vi "Gen Library.vi"(8 "error in (no error)":errorcluster) -> (0 "error out":errorcluster)   [LabVIEW 2020, in "WebServiceImporter.lvlib" / "VI Generator.lvlib"]
uses:
  <vilib>/Platform/WebService/VI Generator/VI Generator.lvlib
  <vilib>/Platform/WebService/Error Handling/Error/Context Name.ctl
  <vilib>/Platform/WebService/Error Handling/Error/Error Number.ctl
  <vilib>/Platform/WebService/Error Handling/Error Handling.lvlib
  <resource>/importtools/Common/LabVIEW Library/NISAST LabVIEW Library.lvlib
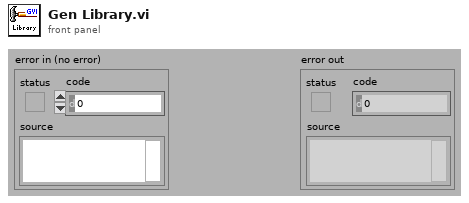
[diagram p1: front panel]
types:
  T1 = typedef "WebServiceImporter.lvlib/Error Handling.lvlib/Error Number.ctl" = u16
  T2 = typedef "WebServiceImporter.lvlib/Error Handling.lvlib/Context Name.ctl" = u16
  T3 = typedef "WebServiceImporter.lvlib/Error Handling.lvlib/Context.ctl" = cluster{"name":T2, "value":string}[]
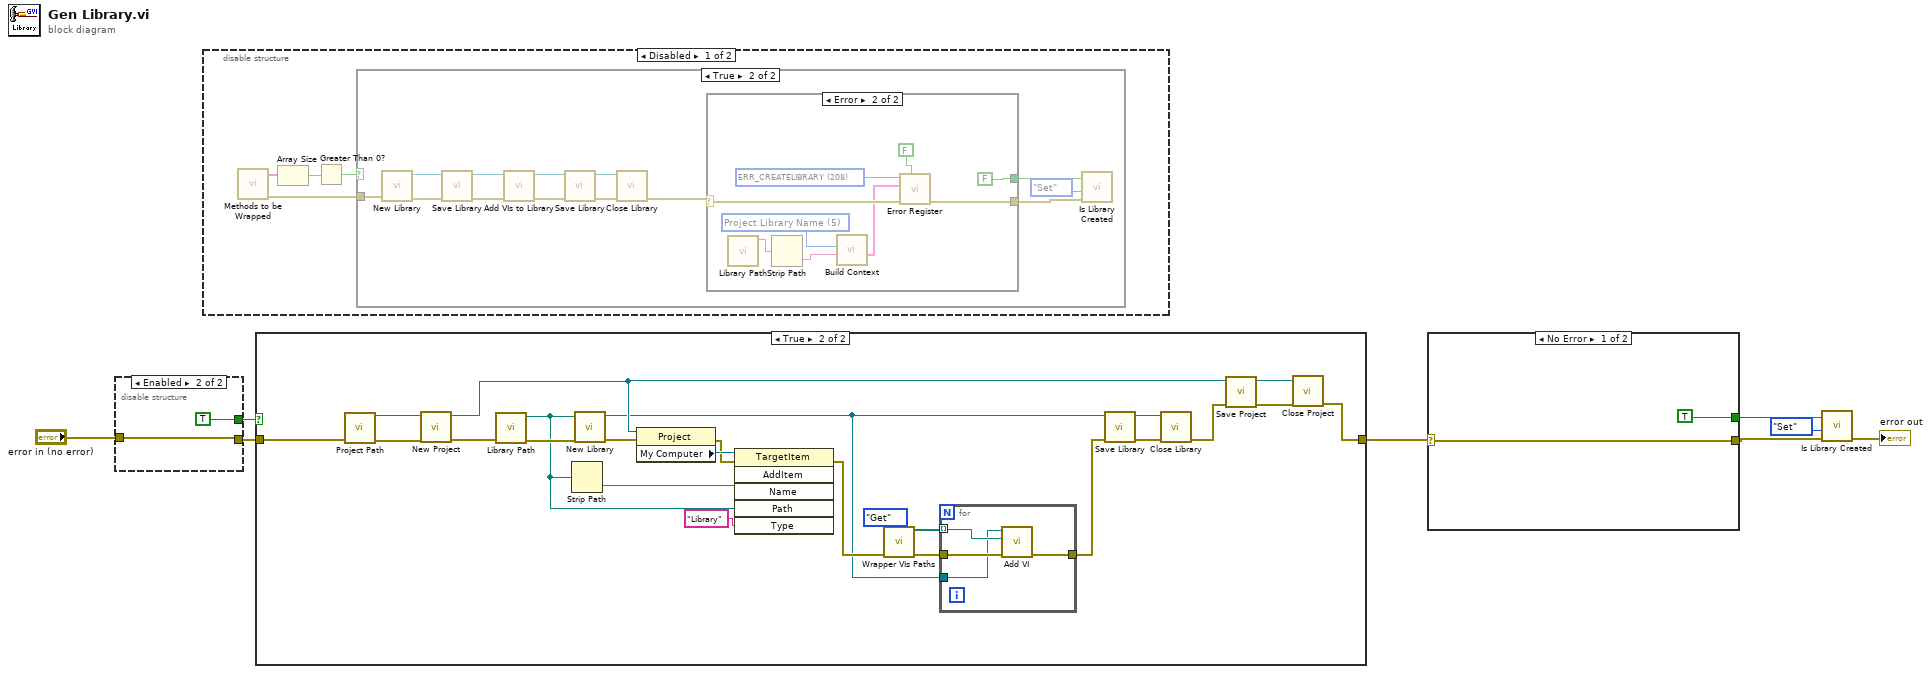
[diagram p0: block diagram]
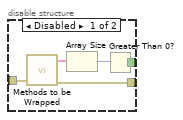
[diagram p2: hidden frame]
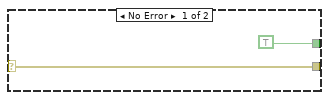
[diagram p4: hidden frame]
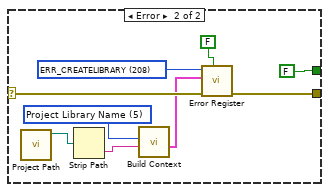
[diagram p6: hidden frame]
diagram:
  n1 = disable-structure shown="Enabled" {
    disable-tunnel: "error in (no error)" -> [w11 w15]
    disable-tunnel: [w10 TRUE] -> w7
    disable-tunnel: [w9 w15] -> w6
    frame Disabled {
      n2 = call <vilib>:"Methods to be Wrapped.vi"("error in (no error)"=w11) -> ("error out"=w9:errorcluster, "Methods to be Wrapped (out)"=w13:string[])  [unwired: 9 in]
      n3 = Array Size(array=w13) -> (size(s)=w12:i32)
      n4 = Greater Than 0?(x=w12) -> (x > 0?=w10:bool)
    }
    frame Enabled {
    }
  }
  n5 = disable-structure shown="Disabled" {
    frame Disabled {
      n6 = call <vilib>:"Methods to be Wrapped.vi"() -> ("error out"=w19:errorcluster, "Methods to be Wrapped (out)"=w16:string[])  [unwired: 10 in]
      n7 = Array Size(array=w16) -> (size(s)=w17:i32)
      n8 = Greater Than 0?(x=w17) -> (x > 0?=w18:bool)
      n9 = case shown="True" w18 {
        tunnel: w19 -> [_ w29]
        frame False {
        }
        frame True {
          n10 = call <vilib>:"New Library.vi"("error in (no error)"=w29) -> ("error out"=w23:errorcluster, "Library:Create"=w21:refnum<vi>)  [unwired: 9 in]
          n11 = call <vilib>:"Save Library.vi"("error in (no error)"=w23, "library"=w21) -> ("error out"=w22:errorcluster, "library out"=w20:refnum<vi>)  [unwired: 8 in]
          n12 = call <vilib>:"Add VIs to Library.vi"("error in"=w22, "Library"=w20) -> ("error out"=w32:errorcluster, "Library out"=w31:refnum<vi>)  [unwired: 8 in]
          n13 = call <vilib>:"Save Library.vi"("error in (no error)"=w32, "library"=w31) -> ("error out"=w25:errorcluster, "library out"=w30:refnum<vi>)  [unwired: 8 in]
          n14 = call <vilib>:"Close Library.vi"("error in (no error)"=w25, "library"=w30) -> ("error out"=w24:errorcluster)  [unwired: 9 in]
          n15 = case shown="Error" w24 {
            selector: w24 -> [w33 w39]
            tunnel: [TRUE FALSE] -> w27
            tunnel: [w33 w36] -> w26
            frame No Error {
            }
            frame Error {
              w37 = T1 208 items=["ERR_NOERROR"=0, "ERR_ACCESS_OUTPUTFOLDER"=1, "ERR_INVALID_LIBRARYNAME"=2, "ERR_CREATE_VIWRAPPER"=3, "ERR_UNKNOWN"=201, "ERR_BAD_ARGUMENT"=202, "ERR_URL_NOTFOUND_BADWSDL"=203, "ERR_BADLYFORMATTEDURL"=204, "ERR_BADHOSTNAME"=205, "ERR_BADDIRECTORY"=206, "ERR_UNAUTHORIZEDACCESS"=207, "ERR_CREATELIBRARY"=208] ("Error Number")
              w42 = T2 5 items=["Method Name", "Parameter Name", "VI Name", "Control Name", "Proxy Dll Path", "Project Library Name"] ("Context Name")
              n16 = call <vilib>:"Library Path.vi"() -> ("Path (out)"=w41:path)  [unwired: 10 in, 1 out]
              n17 = Strip Path(path=w41) -> (name=w40:string)  [unwired: 1 out]
              n18 = call <vilib>:"Build Context.vi"("Context Value"=w40, "Context Name"=w42) -> ("Context"=w38:T3)  [unwired: 9 in]
              n19 = call <vilib>:"Error Register.vi"("Throw Up?"=FALSE, "error in (no error)"=w39, "Context"=w38, "Error Number"=w37) -> ("error out"=w36:errorcluster)  [unwired: 7 in]
            }
          }
          n20 = call <vilib>:"Is Library Created.vi"("error in (no error)"=w26, "Operation"=enum16{"Get", "Set"}."Set", "Created?"=w27) -> ()  [unwired: 7 in, 2 out]
        }
      }
    }
    frame Enabled {
    }
  }
  n21 = case shown="True" w7 {
    tunnel: w6 -> [w44 w49]
    tunnel: [w44 w54] -> w5
    frame False {
    }
    frame True {
      n22 = call <vilib>:"Project Path.vi"("error in (no error)"=w49) -> ("error out"=w51:errorcluster, "Path (out)"=w50:path)  [unwired: 9 in]
      n23 = call <resource>:"New Project.vi"("error in (no error)"=w51, "Path"=w50) -> ("error out"=w52:errorcluster, "new Project"=w60:refnum<vi>)  [unwired: 8 in]
      n24 = call <vilib>:"Library Path.vi"("error in (no error)"=w52) -> ("error out"=w53:errorcluster, "Path (out)"=w47:path)  [unwired: 9 in]
      n25 = Strip Path(path=w47) -> (name=w46:string)  [unwired: 1 out]
      n26 = call <vilib>:"New Library.vi"("error in (no error)"=w53, "Path"=w47) -> ("error out"=w65:errorcluster, "new library"=w45:refnum<vi>)  [unwired: 8 in]
      n27 = property class="Project"(reference=w60, error in=w65) -> (error out=w61:errorcluster, "My Computer"=w64:refnum<vi>)  [unwired: 1 out]
      n28 = invoke class="TargetItem" method="AddItem"(reference=w64, error in=w61, "Name"=w46, "Path"=w47, "Type"="Library") -> (error out=w63:errorcluster)  [unwired: 1 in, 5 out]
      n29 = call <vilib>:"Wrapper VIs Paths.vi"("error in (no error)"=w63, "Op"=enum16{"Get", "Add", "Clear"}."Get") -> ("error out"=w67:errorcluster, "Array"=w66:path[])  [unwired: 8 in]
      n30 = for {
        tunnel: w67 -> [w72]
        tunnel: w66 -> [w71] mode=indexing
        tunnel: w45 -> [w70]
        tunnel: [w69] -> w62
        n31 = call <resource>:"Add VI.vi"("error in (no error)"=w72, "vi path"=w71, "parent"=w70) -> ("error out"=w69:errorcluster)  [unwired: 6 in, 2 out]
      }
      n32 = call <vilib>:"Save Library.vi"("error in (no error)"=w62, "library"=w45) -> ("error out"=w59:errorcluster, "library out"=w58:refnum<vi>)  [unwired: 8 in]
      n33 = call <vilib>:"Close Library.vi"("error in (no error)"=w59, "library"=w58) -> ("error out"=w57:errorcluster)  [unwired: 9 in]
      n34 = call <resource>:"Save Project.vi"("error in (no error)"=w57, "Project"=w60) -> ("error out"=w56:errorcluster, "Project out"=w55:refnum<vi>)  [unwired: 8 in]
      n35 = call <resource>:"Close Project.vi"("error in (no error)"=w56, "Project"=w55) -> ("error out"=w54:errorcluster)  [unwired: 9 in]
    }
  }
  n36 = case shown="No Error" w5 {
    selector: w5 -> [w73 w80]
    tunnel: [TRUE FALSE] -> w3
    tunnel: [w73 w77] -> w2
    frame No Error {
    }
    frame Error {
      w78 = T1 208 items=["ERR_NOERROR"=0, "ERR_ACCESS_OUTPUTFOLDER"=1, "ERR_INVALID_LIBRARYNAME"=2, "ERR_CREATE_VIWRAPPER"=3, "ERR_UNKNOWN"=201, "ERR_BAD_ARGUMENT"=202, "ERR_URL_NOTFOUND_BADWSDL"=203, "ERR_BADLYFORMATTEDURL"=204, "ERR_BADHOSTNAME"=205, "ERR_BADDIRECTORY"=206, "ERR_UNAUTHORIZEDACCESS"=207, "ERR_CREATELIBRARY"=208] ("Error Number")
      w82 = T2 5 items=["Method Name", "Parameter Name", "VI Name", "Control Name", "Proxy Dll Path", "Project Library Name"] ("Context Name")
      n37 = call <vilib>:"Project Path.vi"() -> ("Path (out)"=w75:path)  [unwired: 10 in, 1 out]
      n38 = Strip Path(path=w75) -> (name=w81:string)  [unwired: 1 out]
      n39 = call <vilib>:"Build Context.vi"("Context Value"=w81, "Context Name"=w82) -> ("Context"=w79:T3)  [unwired: 9 in]
      n40 = call <vilib>:"Error Register.vi"("Throw Up?"=FALSE, "error in (no error)"=w80, "Context"=w79, "Error Number"=w78) -> ("error out"=w77:errorcluster)  [unwired: 7 in]
    }
  }
  n41 = call <vilib>:"Is Library Created.vi"("error in (no error)"=w2, "Operation"=enum16{"Get", "Set"}."Set", "Created?"=w3) -> ("error out"=→"error out":errorcluster)  [unwired: 7 in, 1 out]
